vi "GetFocusStatus.vi"(4 "password":string="gamma2018", 6 "Username":string="admin", 7 "HTTP_address":string, 8 "error in (no error)":errorcluster, 10 "Value":T2, 11 "Refnum in":T1) -> (0 "error out":errorcluster, 2 "AuthorizationHeader":string, 3 "headers":string)   [LabVIEW 2016]
uses:
  cgi_string.ctl
  <vilib>/httpClient/ClientHandle.ctl
  <vilib>/httpClient/LabVIEWHTTPClient.lvlib
panel:
  in  "Tab Control":enum32{"Server", "Auth"}(tab)
  out "http:":string
  out "body":string
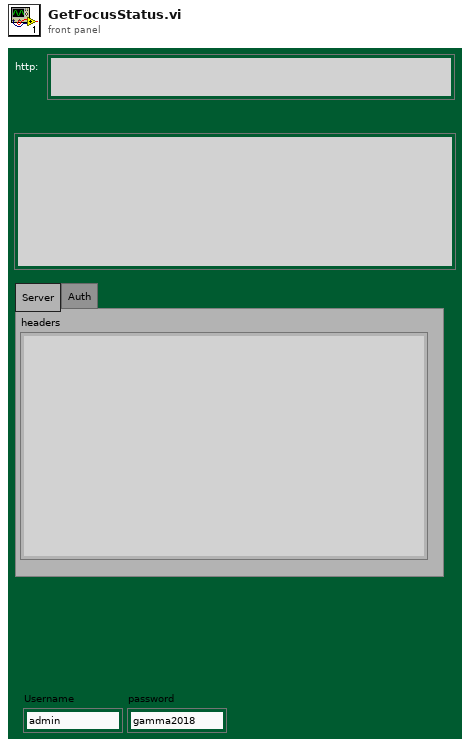
[diagram p1: front panel]
types:
  T1 = typedef "LabVIEWHTTPClient.lvlib/ClientHandle.ctl" = refnum<k1>
  T2 = typedef "cgi_string.ctl" = string
  T3 = cluster{"realm":string, "qop":string, "nounce":string, "opaque":string}
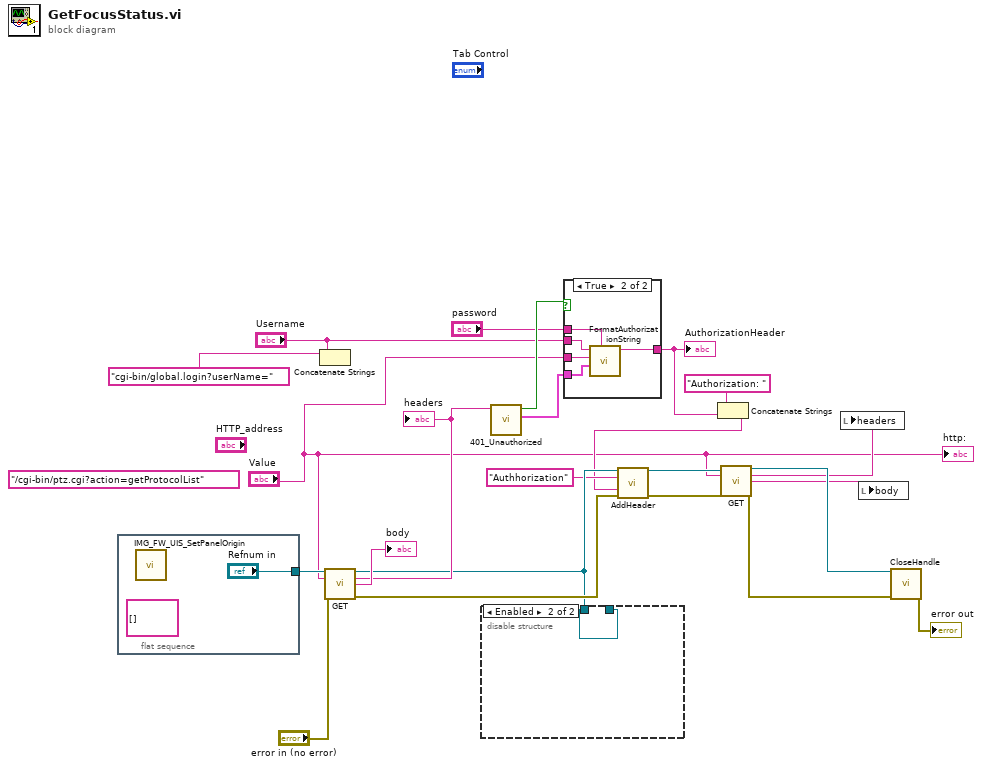
[diagram p0: block diagram]
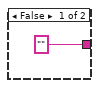
[diagram p2: hidden frame]
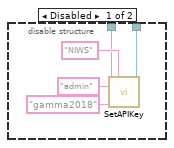
[diagram p3: hidden frame]
diagram:
  (unwired) T2 "/cgi-bin/ptz.cgi?action=getProtocolList" ("Value")
  n1 = flat-sequence {
    tunnel: ["Refnum in"] -> w20
    frame #0 {
      (unwired) string[][] [] ("Table Control")
      n2 = call "IMG_FW_UIS_SetPanelOrigin.vi"() -> ()  [unwired: 11 in, 1 out]
    }
  }
  n3 = Concatenate Strings("cgi-bin/global.login?userName=", "Username") -> ()  [unwired: 1 out]
  n4 = call <vilib>:"GET.vi"("client handle"=w20, "url"="Value", "error in (no error)"="error in (no error)") -> ("client handle out"=w9:T1, "headers"=w16:string, "body"=→"body":string, "error out"=w13:errorcluster)  [unwired: 9 in]
  "headers" <- w16
  n5 = disable-structure shown="Enabled" {
    disable-tunnel: w9 -> [w26 w30]
    disable-tunnel: [w25 w30] -> _
    frame Disabled {
      n6 = call <vilib>:"SetAPIKey.vi"("client handle"=w26, "mode"="NIWS", "access id"="admin", "secret id"="gamma2018") -> ("client handle out"=w25:T1)  [unwired: 10 in, 1 out]
    }
    frame Enabled {
    }
  }
  n7 = call "401_Unauthorized.vi"("headers"=w16) -> ("ServerInfo"=w18:T3, "401?"=w19:bool)  [unwired: 8 in, 1 out]
  n8 = case shown="True" w19 {
    tunnel: w18 -> [_ w36]
    tunnel: "Username" -> [_ w35]
    tunnel: "Value" -> [_ w33]
    tunnel: "password" -> [_ w34]
    tunnel: ["" w32] -> w5
    frame False {
    }
    frame True {
      n9 = call "FormatAuthorizationString.vi"("password"=w34, "ServerInfo"=w36, "String in"=w33, "Username"=w35) -> ("String out"=w32:string)  [unwired: 7 in]
    }
  }
  "AuthorizationHeader" <- w5
  n10 = Concatenate Strings("Authorization: " ("string"), w5) -> (w2:string)
  n11 = call <vilib>:"AddHeader.vi"("client handle"=w9, "header"="Authhorization" ("access id"), "value"=w2, "error in (no error)"=w13) -> ("client handle out"=w4:T1, "error out"=w3:errorcluster)  [unwired: 10 in]
  n12 = call <vilib>:"GET.vi"("client handle"=w4, "url"="Value", "error in (no error)"=w3) -> ("client handle out"=w14:T1, "headers"=w10:string, "body"=w11:string, "error out"=w12:errorcluster)  [unwired: 9 in]
  n13 = local write "headers"(w10) -> ()
  n14 = local write "body"(w11) -> ()
  n15 = call <vilib>:"CloseHandle.vi"("client handle"=w14, "error in (no error)"=w12) -> ("error out"=→"error out":errorcluster)  [unwired: 13 in]
  "http:" <- "Value"
